vi "Config - Read Data.vi"(8 "error in (no error)":errorcluster) -> (0 "error out":errorcluster, 2 "Data Record":T1)   [LabVIEW 2017]
doc: "Reads configuration data record from external XML file."
uses:
  Controls/Config Data Record.ctl
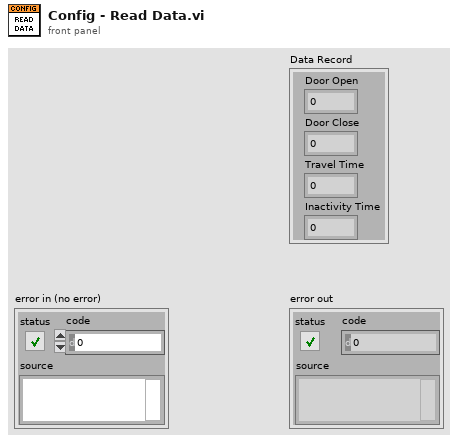
[diagram p1: front panel]
types:
  T1 = typedef "Config Data Record.ctl" = cluster{"Door Open":dbl, "Door Close":dbl, "Travel Time":dbl, "Inactivity Time":dbl}
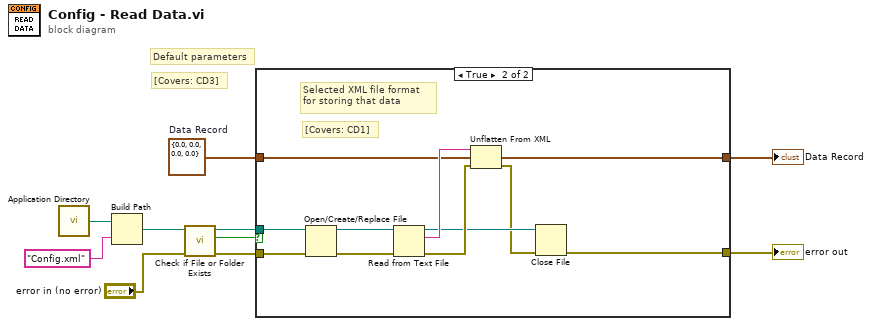
[diagram p0: block diagram]
diagram:
  w7 = T1 {"Door Open"=0.0, "Door Close"=0.0, "Travel Time"=0.0, "Inactivity Time"=0.0}  # Data Record
  # "[Covers: CD3]"
  # "Default parameters"
  n1 = call <vilib>:"Application Directory.vi"() -> ("Application Directory"=w10:path)
  n2 = Build Path(base path=w10, name or relative path="Config.xml") -> (appended path=w8:path)
  n3 = call <vilib>:"Check if File or Folder Exists.vi"("error in (no error)"="error in (no error)", "path"=w8) -> ("error out"=w4:errorcluster, "file or folder exists?"=w6:bool, "dup path"=w5:path)  [unwired: 7 in]
  n4 = case shown="True" w6 {
    tunnel: w7 -> [w12 w18]
    tunnel: w5 -> [_ w22]
    tunnel: w4 -> [w11 w23]
    tunnel: [w12 w14] -> w3
    tunnel: [w11 w13] -> w2
    frame False {
      # "[Covers: CD3]"
    }
    frame True {
      # "[Covers: CD1]"
      # "Selected XML file format \nfor storing that data"
      n5 = Open/Create/Replace File(file path (use dialog)=w22, error in=w23) -> (refnum out=w20:refnum<file>, error out=w21:errorcluster)  [unwired: 4 in, 1 out]
      n6 = Read from Text File(file (use dialog)=w20, error in=w21) -> (refnum out=w16:refnum<file>, text=w19:string, error out=w17:errorcluster)  [unwired: 2 in, 1 out]
      n7 = Unflatten From XML(xml string=w19, type=w18, error in (no error)=w17) -> (value=w14:T1, error out=w15:errorcluster)
      n8 = Close File(refnum=w16, error in=w15) -> (error out=w13:errorcluster)  [unwired: 1 out]
    }
  }
  "error out" <- w2
  "Data Record" <- w3
